vi "ShooterFuncGlob.vi"(10 "Operation":T15, 11 "ShooterDevRefIn":T1={"Wench Motor"={"DeviceStatus"={"status"=FALSE, "code"=0, "source"=""}, "Type"=enum."PWM", "PWM"={"Digital Module"=enum."Digital Module 1", "PWM Channel"=enum."Invalid", "DeadBand"={"Name"="", "maxPositivePwm"=0, "minPositivePwm"=0, "centerPwm"=0, "maxNegativePwm"=0, "minNegativePwm"=0, "angularRange"=0}}, "CAN"={"Device Number"=0, "Control Mode"=enum."Percent VBus", "Semaphore"=refnum, "Max Vout"=12.0}, "Invert"=FALSE, "TransformRef"=refnum, "InvTransformRef"=refnum}, "Lower Wench Limit"={"DevStatus"={"status"=FALSE, "code"=0, "source"=""}, "DIO Channel"=enum."DIO 1", "Digital Module"=enum."Digital Module 1"}, "Clutch Engaged Sensor"={"DevStatus"={"status"=FALSE, "code"=0, "source"=""}, "DIO Channel"=enum."DIO 1", "Digital Module"=enum."Digital Module 1"}, "Wench Encoder"={"DevStatus"={"status"=FALSE, "code"=0, "source"=""}, "EncoderIndex"=enum."Invalid", "CounterIndex"=enum."Invalid", "DistancePerCount"=1.0, "Decoding Type"=enum."4x"}, "Worm Motor"={"DeviceStatus"={"status"=FALSE, "code"=0, "source"=""}, "Type"=enum."PWM", "PWM"={"Digital Module"=enum."Digital Module 1", "PWM Channel"=enum."Invalid", "DeadBand"={"Name"="", "maxPositivePwm"=0, "minPositivePwm"=0, "centerPwm"=0, "maxNegativePwm"=0, "minNegativePwm"=0, "angularRange"=0}}, "CAN"={"Device Number"=0, "Control Mode"=enum."Percent VBus", "Semaphore"=refnum, "Max Vout"=12.0}, "Invert"=FALSE, "TransformRef"=refnum, "InvTransformRef"=refnum}, "Worm Screw Out Sensor"={"DevStatus"={"status"=FALSE, "code"=0, "source"=""}, "DIO Channel"=enum."DIO 1", "Digital Module"=enum."Digital Module 1"}, "Clutch Disengaged Sensor"={"DevStatus"={"status"=FALSE, "code"=0, "source"=""}, "DIO Channel"=enum."DIO 1", "Digital Module"=enum."Digital Module 1"}}) -> (3 "ShooterDevRefOut":T1={"Wench Motor"={"DeviceStatus"={"status"=FALSE, "code"=0, "source"=""}, "Type"=enum."PWM", "PWM"={"Digital Module"=enum."Digital Module 1", "PWM Channel"=enum."Invalid", "DeadBand"={"Name"="", "maxPositivePwm"=0, "minPositivePwm"=0, "centerPwm"=0, "maxNegativePwm"=0, "minNegativePwm"=0, "angularRange"=0}}, "CAN"={"Device Number"=0, "Control Mode"=enum."Percent VBus", "Semaphore"=refnum, "Max Vout"=12.0}, "Invert"=FALSE, "TransformRef"=refnum, "InvTransformRef"=refnum}, "Lower Wench Limit"={"DevStatus"={"status"=FALSE, "code"=0, "source"=""}, "DIO Channel"=enum."DIO 1", "Digital Module"=enum."Digital Module 1"}, "Clutch Engaged Sensor"={"DevStatus"={"status"=FALSE, "code"=0, "source"=""}, "DIO Channel"=enum."DIO 1", "Digital Module"=enum."Digital Module 1"}, "Wench Encoder"={"DevStatus"={"status"=FALSE, "code"=0, "source"=""}, "EncoderIndex"=enum."Invalid", "CounterIndex"=enum."Invalid", "DistancePerCount"=1.0, "Decoding Type"=enum."4x"}, "Worm Motor"={"DeviceStatus"={"status"=FALSE, "code"=0, "source"=""}, "Type"=enum."PWM", "PWM"={"Digital Module"=enum."Digital Module 1", "PWM Channel"=enum."Invalid", "DeadBand"={"Name"="", "maxPositivePwm"=0, "minPositivePwm"=0, "centerPwm"=0, "maxNegativePwm"=0, "minNegativePwm"=0, "angularRange"=0}}, "CAN"={"Device Number"=0, "Control Mode"=enum."Percent VBus", "Semaphore"=refnum, "Max Vout"=12.0}, "Invert"=FALSE, "TransformRef"=refnum, "InvTransformRef"=refnum}, "Worm Screw Out Sensor"={"DevStatus"={"status"=FALSE, "code"=0, "source"=""}, "DIO Channel"=enum."DIO 1", "Digital Module"=enum."Digital Module 1"}, "Clutch Disengaged Sensor"={"DevStatus"={"status"=FALSE, "code"=0, "source"=""}, "DIO Channel"=enum."DIO 1", "Digital Module"=enum."Digital Module 1"}})   [LabVIEW 2013]
uses:
  Utils/GetSetType.ctl
  Utils/ShooterDevRef.ctl
  <vilib>/Rock Robotics/WPI/MotorControl/WPI_MotorControlDeviceRef.ctl
  <vilib>/Rock Robotics/SystemInterfaces/Typedef/FPGA_TypedefDigitalModule.ctl
  <vilib>/Rock Robotics/SystemInterfaces/DIO/FPGA_DIOPWMChannel.ctl
  <vilib>/Rock Robotics/WPI/PWM/WPI_PWMDeadband.ctl
  <vilib>/Rock Robotics/WPI/CAN/Jaguar/SubVIs/WPI_CANJaguar_ControlMode.ctl
  <vilib>/Rock Robotics/WPI/PWM/WPI_PWMTransform_ConPane.ctl
  <vilib>/Rock Robotics/WPI/DigitalInput/WPI_DigitalInputDevRef.ctl
  <vilib>/Rock Robotics/SystemInterfaces/DIO/FPGA_DIOChannel.ctl
  <vilib>/Rock Robotics/WPI/Encoder/WPI_EncoderDevRef.ctl
  <vilib>/Rock Robotics/SystemInterfaces/Encoder/FPGA_EncoderIdx.ctl
  <vilib>/Rock Robotics/SystemInterfaces/Counter/FPGA_CounterCtrSystemIndex.ctl
  <vilib>/Rock Robotics/WPI/Encoder/WPI_EncoderType.ctl
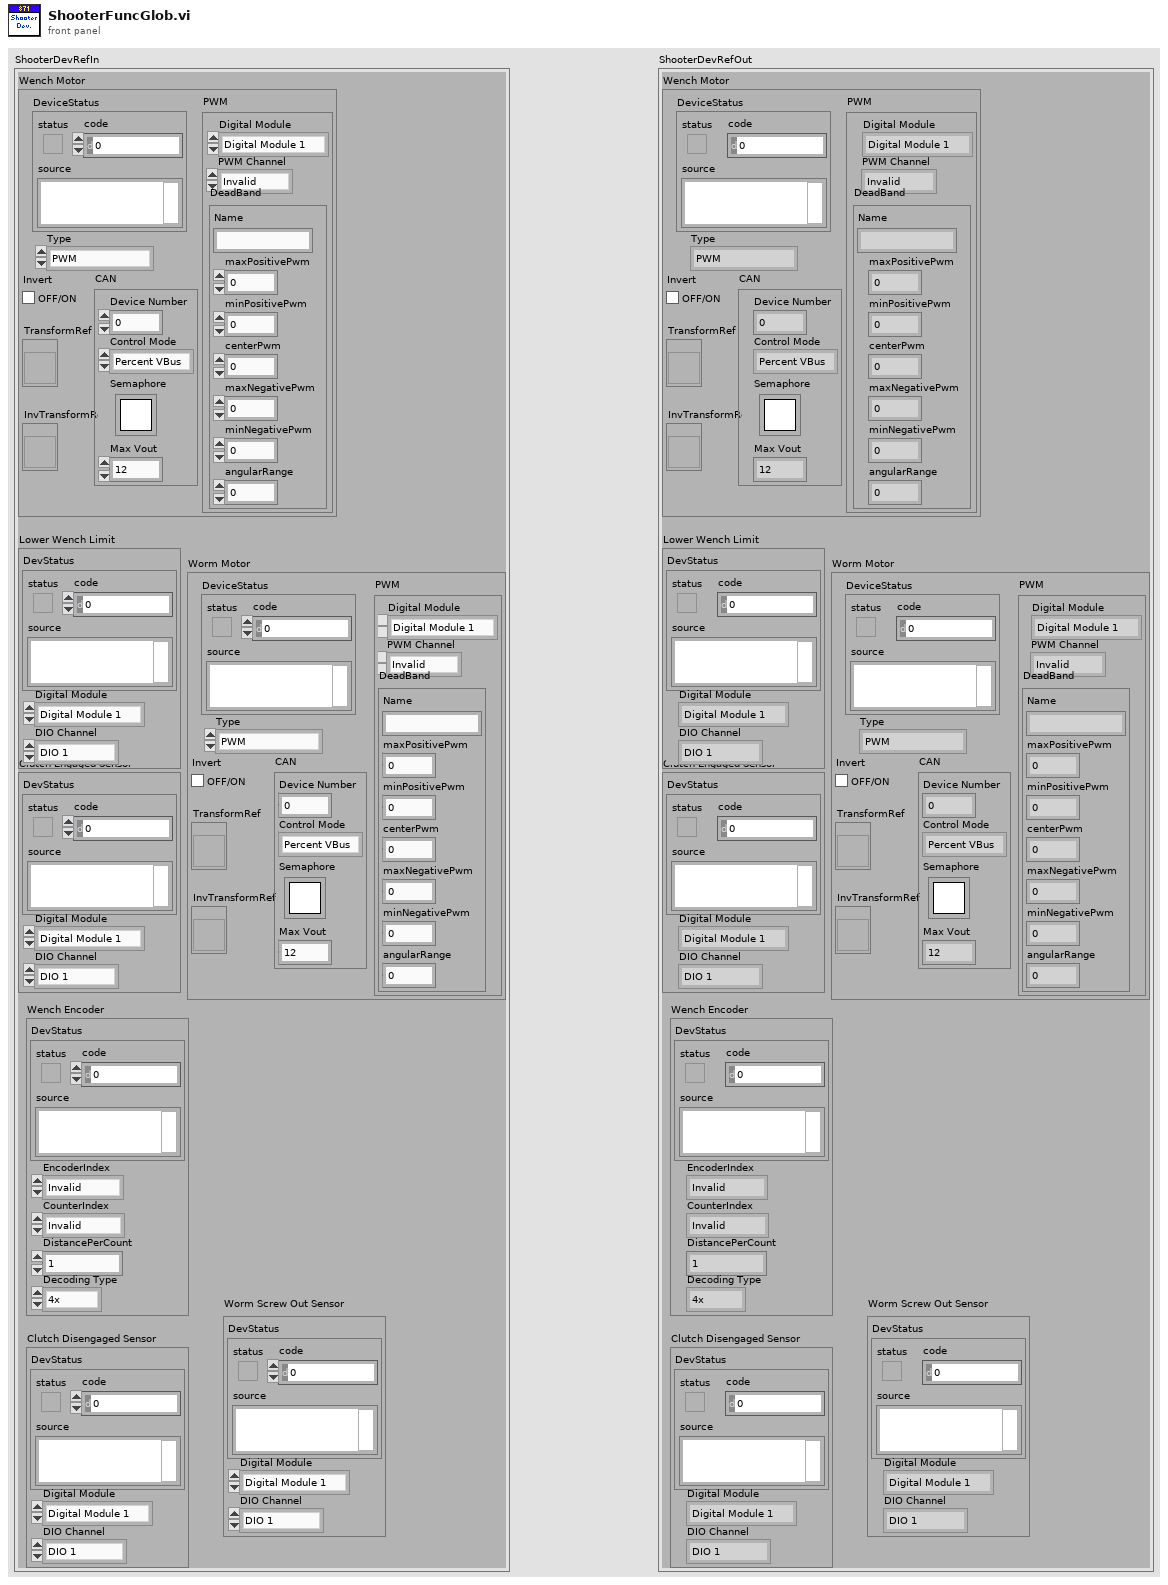
[diagram p1: front panel]
types:
  T1 = typedef "ShooterDevRef.ctl" = cluster{"Wench Motor":T2, "Lower Wench Limit":T9, "Clutch Engaged Sensor":T9, "Wench Encoder":T11, "Worm Motor":T2, "Worm Screw Out Sensor":T9, "Clutch Disengaged Sensor":T9}
  T2 = typedef "WPI_MotorControlDeviceRef.ctl" = cluster{"DeviceStatus":errorcluster, "Type":enum16{"PWM", "CAN"}, "PWM":cluster{"Digital Module":T3, "PWM Channel":T4, "DeadBand":T5}, "CAN":cluster{"Device Number":u8, "Control Mode":T6, "Semaphore":T7, "Max Vout":dbl}, "Invert":bool, "TransformRef":T8, "InvTransformRef":T8}
  T3 = typedef "FPGA_TypedefDigitalModule.ctl" = enum16{"Digital Module 1", "Digital Module 2"}
  T4 = typedef "FPGA_DIOPWMChannel.ctl" = enum8{"PWM 1", "PWM 2", "PWM 3", "PWM 4", "PWM 5", "PWM 6", "PWM 7", "PWM 8", "PWM 9", "PWM 10", "Invalid"}
  T5 = typedef "WPI_PWMDeadband.ctl" = cluster{"Name":string, "maxPositivePwm":i32, "minPositivePwm":i32, "centerPwm":i32, "maxNegativePwm":i32, "minNegativePwm":i32, "angularRange":u16}
  T6 = typedef "WPI_CANJaguar_ControlMode.ctl" = enum8{"Percent VBus", "Current", "Speed", "Position", "Voltage"}
  T7 = typedef "Semaphore RefNum" = refnum<k1>
  T8 = typedef "WPI_PWMTransform_ConPane.ctl" = refnum<vi>
  T9 = typedef "WPI_DigitalInputDevRef.ctl" = cluster{"DevStatus":errorcluster, "DIO Channel":T10, "Digital Module":T3}
  T10 = typedef "FPGA_DIOChannel.ctl" = enum8{"DIO 1", "DIO 2", "DIO 3", "DIO 4", "DIO 5", "DIO 6", "DIO 7", "DIO 8", "DIO 9", "DIO 10", "DIO 11", "DIO 12", "DIO 13", "DIO 14", "Invalid"}
  T11 = typedef "WPI_EncoderDevRef.ctl" = cluster{"DevStatus":errorcluster, "EncoderIndex":T12, "CounterIndex":T13, "DistancePerCount":dbl, "Decoding Type":T14}
  T12 = typedef "FPGA_EncoderIdx.ctl" = enum8{"Enc 0", "Enc 1", "Enc 2", "Enc 3", "Invalid"}
  T13 = typedef "FPGA_CounterCtrSystemIndex.ctl" = enum8{"Ctr 0", "Ctr 1", "Ctr 2", "Ctr 3", "Ctr 4", "Ctr 5", "Ctr 6", "Ctr 7", "Invalid"}
  T14 = typedef "WPI_EncoderType.ctl" = enum16{"1x", "2x", "4x"}
  T15 = typedef "GetSetType.ctl" = enum16{"Get", "Set"}
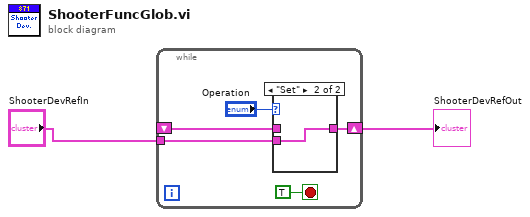
[diagram p0: block diagram]
diagram:
  n1 = while {
    shift-right: [w5] -> w1
    shift-left: _ -> [w4]
    tunnel: "ShooterDevRefIn" -> [w3]
    stop <- TRUE stop-if-true
    n2 = case shown="\"Set\"" "Operation" {
      tunnel: w3 -> [_ w9]
      tunnel: [w8 w9] -> w5
      tunnel: w4 -> [w8 _]
      frame "Get", Default {
      }
      frame "Set" {
      }
    }
  }
  "ShooterDevRefOut" <- w1
